vi "buildSetTemperature.vi"(8 "error in (no error)":errorcluster, 10 "temperature[°C]":i32, 11 "PlainTextCommandBuilder in":refnum<class "XMLCommandBuilder.lvclass">) -> (0 "error out":errorcluster, 2 "message":string, 3 "PlainTextCommandBuilder out":refnum<class "XMLCommandBuilder.lvclass">)   [LabVIEW 2023, in "AbstractFactory.lvlib" / "XMLCommandBuilder.lvclass"]
uses:
  XMLCommandBuilder.lvclass
  XMLCommandBuilder.lvclass/XMLCommandBuilder.ctl
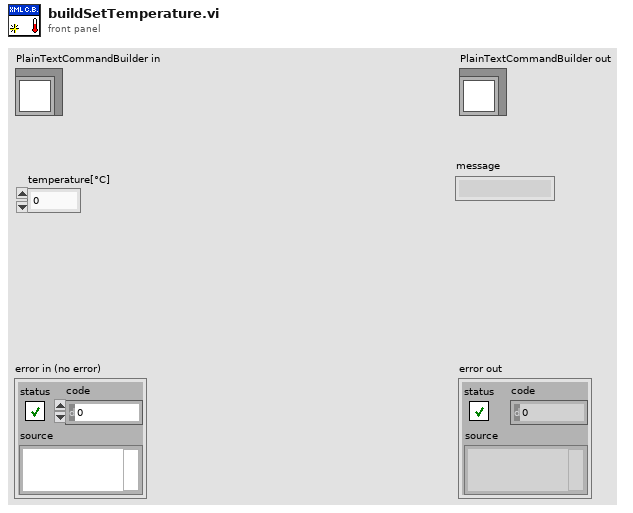
[diagram p1: front panel]
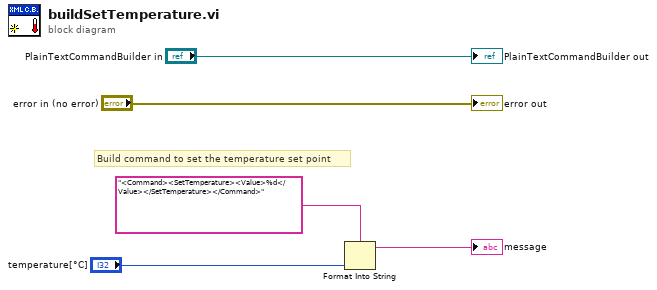
[diagram p0: block diagram]
diagram:
  # "Build command to set the temperature set point"
  n1 = Format Into String(format string="<Command><SetTemperature><Value>%d</Value></SetTemperature></Command>", "temperature[°C]") -> (resulting string=→"message":string)  [unwired: 2 in, 1 out]
  "error out" <- "error in (no error)"
  "PlainTextCommandBuilder out" <- "PlainTextCommandBuilder in"
